vi "delete tree item.vi"(8 "error in":errorcluster, 10 "Tag":string, 11 "tree reference in":refnum<vi>) -> (0 "error out":errorcluster, 3 "tree reference out":refnum<vi>)   [LabVIEW 2015, in "TDMS datalogger editor node.lvclass"]
uses:
  TDMS datalogger editor node.lvclass
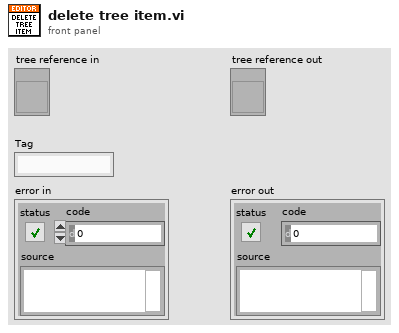
[diagram p1: front panel]
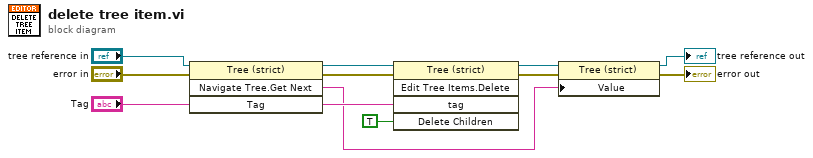
[diagram p0: block diagram]
diagram:
  n1 = invoke class="Tree (strict)" method="Navigate Tree.Get Next"(reference="tree reference in", error in="error in", "Tag"="Tag") -> (reference out=w4:refnum<vi>, error out=w5:errorcluster, "Navigate Tree:Get Next Item"=w3:string)  [unwired: 1 in, 1 out]
  n2 = invoke class="Tree (strict)" method="Edit Tree Items.Delete"(reference=w4, error in=w5, "tag"="Tag", "Delete Children"=TRUE ("Delete Children?")) -> (reference out=w1:refnum<vi>, error out=w2:errorcluster)  [unwired: 1 in, 3 out]
  n3 = property class="Tree (strict)"(reference=w1, error in=w2, "Value"=w3) -> (reference out=→"tree reference out":refnum<vi>, error out=→"error out":errorcluster)
